vi "ArmStates.vi"(10 "Fuel Arm":bool, 11 "Arm":bool) -> (0 "All\nSolenoids":bool[](array[boolean]))   [LabVIEW 2016]
panel:
  out "Time Elapsed":dbl
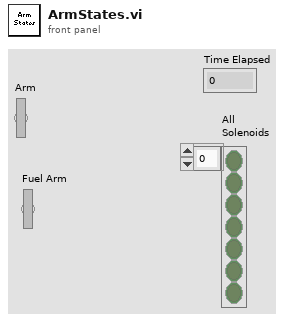
[diagram p1: front panel]
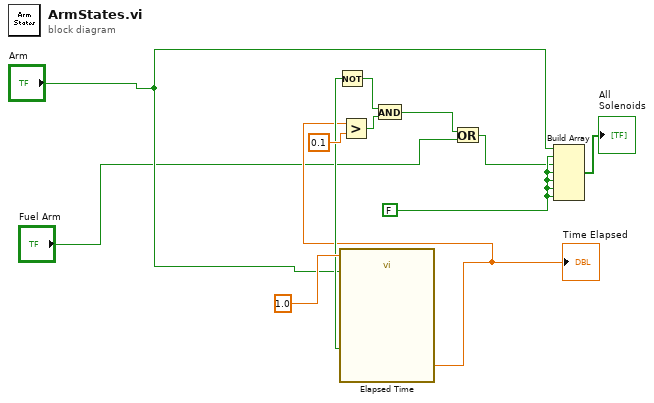
[diagram p0: block diagram]
diagram:
  w10 = FALSE ("Arm")
  n1 = call "Elapsed Time"("Time Target (s)"=1.0, "Reset"="Arm") -> ("Elapsed Time (s)"=w5:dbl, "Time has Elapsed"=w6:bool)  [unwired: 10 in, 6 out]
  "Time Elapsed" <- w5
  n2 = Not(x=w6) -> (.not. x?=w7:bool)
  n3 = Greater?(x=w5, y=0.1) -> (0:w8:bool)
  n4 = And(x=w7, y=w8) -> (x .and. y?=w3:bool)
  n5 = Or(x=w3, y="Fuel Arm") -> (x .or. y?=w1:bool)
  n6 = Build Array("Arm", w10, w1, w10, w10, w10, w10) -> (→"All\nSolenoids":bool[])
